vi "chart_vs_graph.vi"() -> ()   [LabVIEW 2022 SP3]
panel:
  out "Waveform Graph":dbl[](graph)
  out "Waveform Chart":dbl(graph)
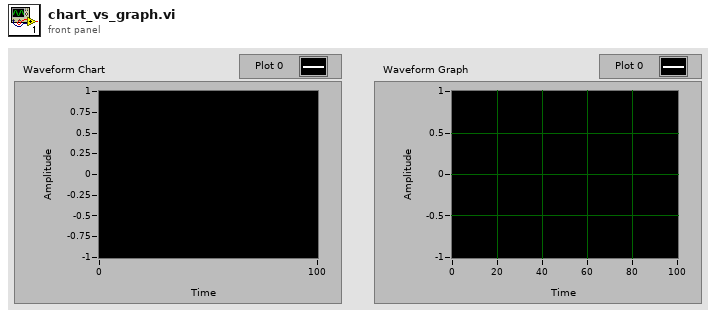
[diagram p1: front panel]
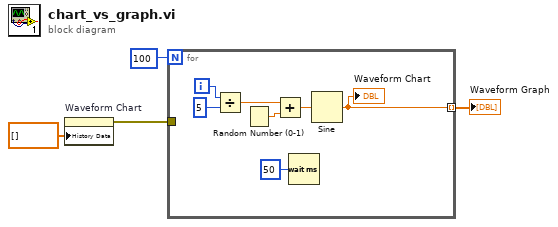
[diagram p0: block diagram]
diagram:
  n1 = property on="Waveform Chart" class="WFChart (严格)"("History Data"=dbl[] []) -> (error out=w1:errorcluster)  [unwired: 2 in, 1 out]
  n2 = for {
    N: 100 -> [_]
    tunnel: [w10] -> w3 mode=indexing
    tunnel: w1 -> [_]
    i -> [w11]
    n3 = Divide(x=w11, y=5) -> (x/y=w8:dbl)
    n4 = Random Number (0-1)() -> (number: 0 to 1=w9:dbl)
    n5 = Add(x=w8, y=w9) -> (x+y=w7:dbl)
    n6 = Wait (ms)(milliseconds to wait=u32 50) -> ()  [unwired: 1 out]
    n7 = Sine(x=w7) -> (sin(x)=w10:dbl)
    "Waveform Chart" <- w10
  }
  "Waveform Graph" <- w3
